vi "minmax_scale.vi"(8 "error in":errorcluster caption="entrée d'erreur", 10 "X":string[][](array[string]), 11 "minmax_scale":T2={"feature_range"={"min"=0.0, "max"=1.0}, "axis"=0, "copy"=TRUE}) -> (0 "error out":errorcluster caption="sortie d'erreur", 3 "Data":T1)   [LabVIEW 2020]
doc: "Transform features by scaling each feature to a given range.\n\nThis estimator scales and translates each feature individually such that it is in the given range on the training set, i.e. between zero and one.\n\nThe transformation is given by (when axis=0) :\n\nX_std = (X - X.min(axis=0)) / (X.max(axis=0) - X.min(axis=0))\nX_scaled = X_std * (max - min) + min\n\nwhere min, max = feature_range.\n\nThe transformation is calculated as (when axis=0) :\n\nX_scaled = scale * X + min - X.min(axis=0) * scale\nwhere scale = (max - min) / (X.max(axis=0) - X.min(axis=0))\n\nThis transformation is often used as an alternative to zero mean, unit variance scaling.\n\nParameters :\n\n- X : array-like of shape (n_samples, n_features)\nThe data.\n\n- feature_range : tuple (min, max), default=(0, 1)\nDesired range of transformed data.\n\n- axis : int, default=0\nAxis used to scale along. If 0, independently scale each feature, otherwise (if 1) scale each sample.\n\n- copy : bool, default=True\nSet to False to perform inplace scaling and avoid a copy (if the input is already a numpy array)."
uses:
  minmax_scale.lvclass
panel:
  out "minmax_scale.lvclass":refnum<class "minmax_scale.lvclass">
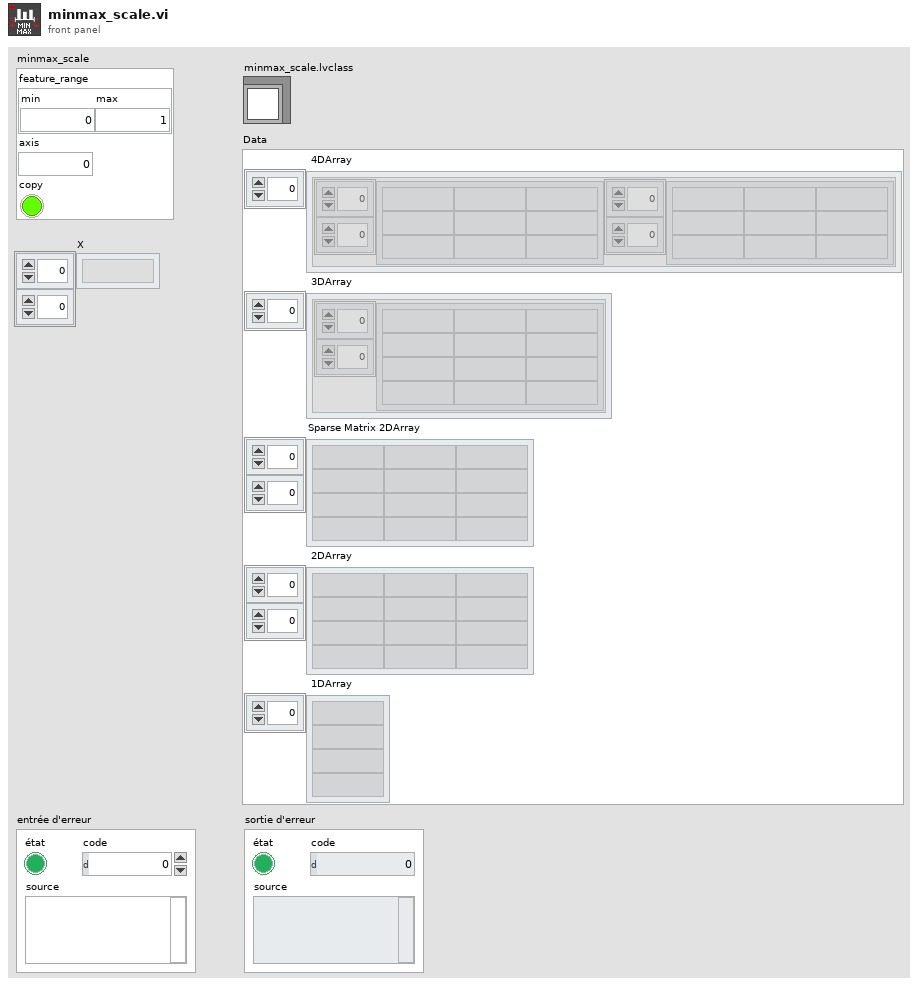
[diagram p1: front panel]
types:
  T1 = cluster{" 4DArray":cluster{"1":string[][], "2":string[][]}[], " 3DArray":cluster{"Tableau":string[][]}[], "Sparse Matrix 2DArray":string[][], " 2DArray":string[][], " 1DArray":string[]}
  T2 = cluster{"feature_range":cluster{"min":dbl, "max":dbl}, "axis":i32, "copy":bool}
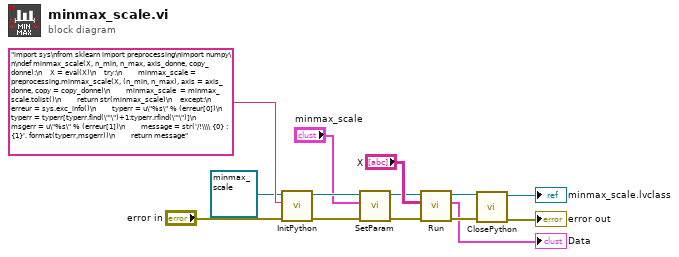
[diagram p0: block diagram]
diagram:
  n1 = call-dynamic "InitPython.vi"("error in (no error)"="error in", "Python Instruction"="import sys\nfrom sklearn import preprocessing\nimport numpy\n\ndef minmax_scale(X, n_min, n_max, axis_donne, copy_donne):\n    X = eval(X)\n    try:\n        minmax_scale = preprocessing.minmax_scale(X, (n_min, n_max), axis = axis_donne, copy = copy_donne)\n        minmax_scale  = minmax_scale.tolist()\n        return str(minmax_scale)\n    except:\n        erreur = sys.exc_info()\n        typerr = u\"%s\" % (erreur[0])\n        typerr = typerr[typerr.find(\"'\")+1:typerr.rfind(\"'\")]\n        msgerr = u\"%s\" % (erreur[1])\n        message = str('/!\\\\ {0} : {1}'. format(typerr,msgerr))\n        return message", "Scikit-learn en entrée"=refnum<class "minmax_scale.lvclass"> refnum ("minmax_scale.lvclass")) -> ("error out"=w3:errorcluster, "Scikit-learn en sortie"=w5:refnum<class "minmax_scale.lvclass">)  [unwired: 7 in]
  n2 = call "SetParam.vi"("error in (no error)"=w3, "minmax_scale"="minmax_scale", "minmax_scale.lvclass"=w5) -> ("error out"=w2:errorcluster, "minmax_scale.lvclass"=w1:refnum<class "minmax_scale.lvclass">)  [unwired: 7 in]
  n3 = call-dynamic "Run.vi"("error in (no error)"=w2, "X"="X", "minmax_scale.lvclass"=w1) -> ("error out"=w9:errorcluster, "Data"=→"Data":T1, "minmax_scale.lvclass"=w10:refnum<class "minmax_scale.lvclass">)  [unwired: 6 in]
  n4 = call-dynamic "ClosePython.vi"("error in (no error)"=w9, "Scikit-learn en entrée"=w10) -> ("error out"=→"error out":errorcluster, "Scikit-learn en sortie"=→"minmax_scale.lvclass":refnum<class "minmax_scale.lvclass">)  [unwired: 8 in]
